vi "Set Script Characteristic.vi"(7 "Script Name":string, 8 "error in (no error)":errorcluster, 9 "Auto Run (F: Disable)":bool, 10 "Script Variable":string, 11 "VISA resource name":refnum<visa-resource-name>) -> (0 "error out":errorcluster, 3 "VISA resource name out":refnum<visa-resource-name>)   [LabVIEW 2017, in "Keithley 2600 Series.lvlib"]
doc: "Configures the script characteristic."
uses:
  <instrlib>/Keithley 2600 Series/Keithley 2600 Series.lvlib
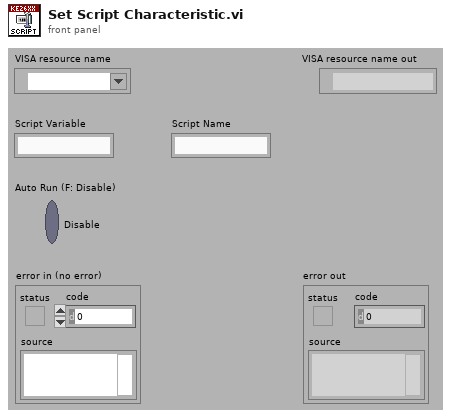
[diagram p1: front panel]
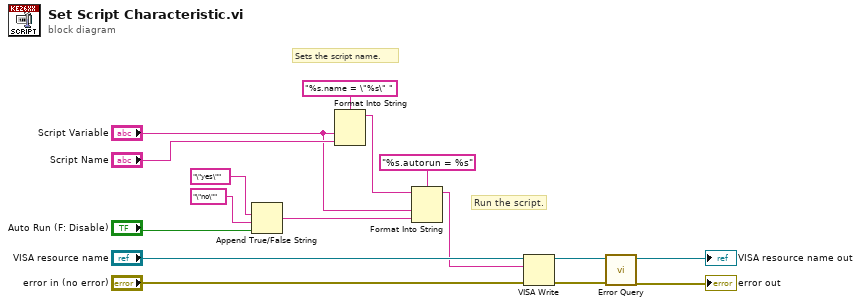
[diagram p0: block diagram]
diagram:
  # "Run the script."
  # "Sets the script name."
  n1 = Append True/False String(1:"Auto Run (F: Disable)", 2:"\"no\"", 3:"\"yes\"") -> (0:w4:string)  [unwired: 1 in]
  n2 = Format Into String(format string="%s.name = \"%s\" ", "Script Variable", "Script Name") -> (resulting string=w2:string)  [unwired: 2 in, 1 out]
  n3 = Format Into String(format string="%s.autorun = %s", initial string=w2, "Script Variable", w4) -> (resulting string=w1:string)  [unwired: 1 in, 1 out]
  n4 = VISA Write(VISA resource name="VISA resource name", write buffer=w1, error in (no error)="error in (no error)") -> (VISA resource name out=w9:refnum<visa-resource-name>, error out=w8:errorcluster)  [unwired: 1 out]
  n5 = call <instrlib>:"Error Query.vi"("error in (no error)"=w8, "VISA resource name"=w9) -> ("error out"=→"error out":errorcluster, "VISA resource name out"=→"VISA resource name out":refnum<visa-resource-name>)  [unwired: 6 in, 2 out]
